vi "Logging Settings Session.vi"(0 "Type":enum16{"Set Settings", "Get Settings"}(ring)=enum."Get Settings", 11 "Error In":errorcluster) -> (6 "Logging Settings":T1={"Logging Interval [s]"=1.0, "Use Lowpass Filter"=TRUE, "Tf [s]"=5.0, "Logging Data to File"=TRUE, "Log Folder"=path "c:/Temp/Data.lvm", "Logging Data to Cloud Service"=FALSE, "Data Cloud Service Url"="http://127.0.0.1:8001/DataWS", "Use Random Data"=TRUE}, 15 "Error Out":errorcluster)   [LabVIEW 2019]
uses:
  Controls/Logging Settings.ctl
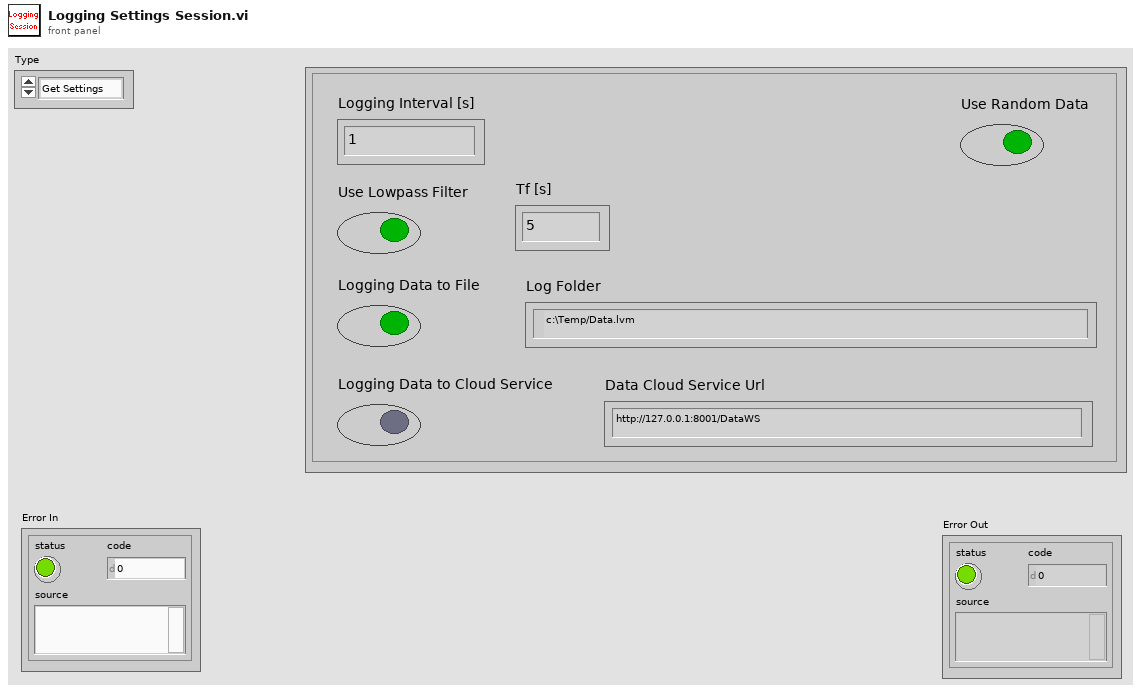
[diagram p1: front panel]
types:
  T1 = typedef "Logging Settings.ctl" = cluster{"Logging Interval [s]":dbl, "Use Lowpass Filter":bool, "Tf [s]":dbl, "Logging Data to File":bool, "Log Folder":path, "Logging Data to Cloud Service":bool, "Data Cloud Service Url":string, "Use Random Data":bool}
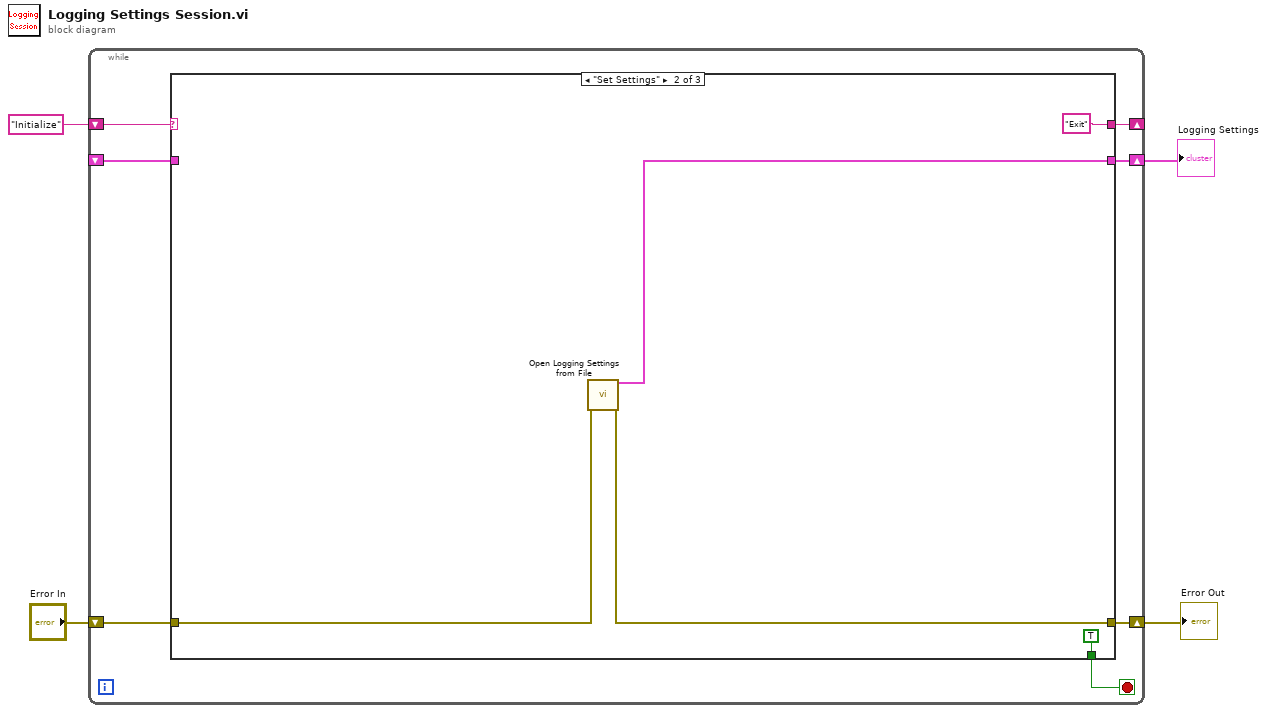
[diagram p0: block diagram]
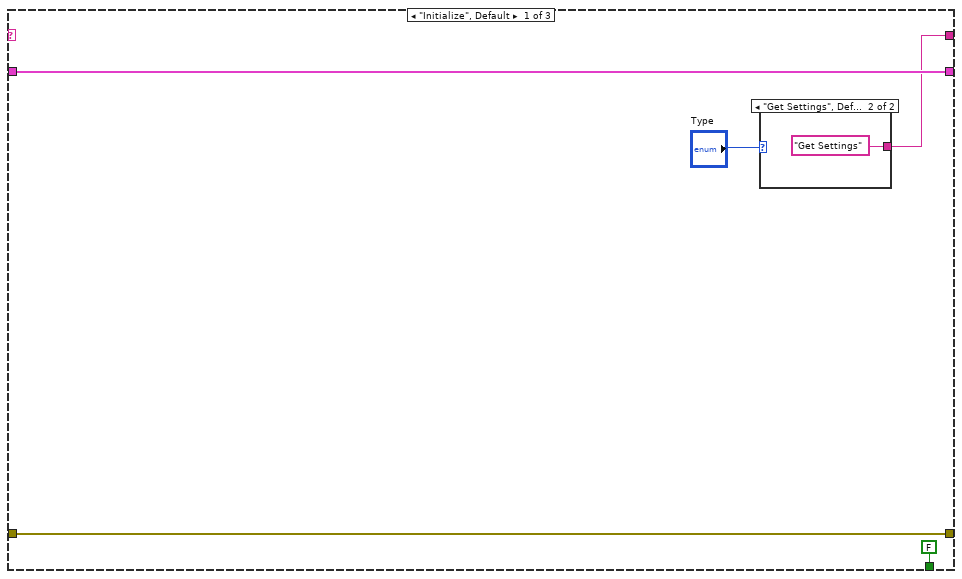
[diagram p2: hidden frame]
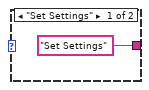
[diagram p3: hidden frame]
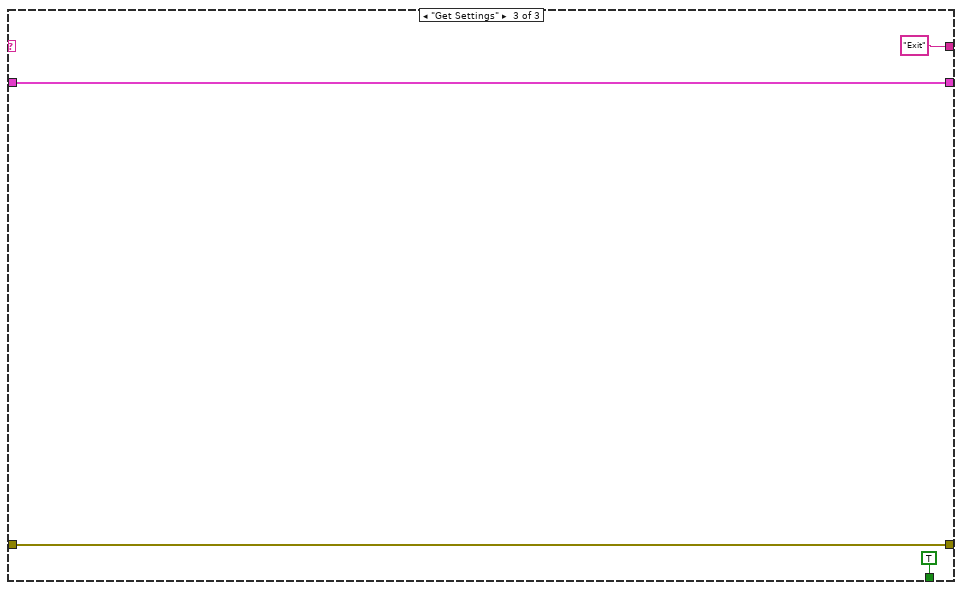
[diagram p4: hidden frame]
diagram:
  n1 = while {
    shift-right: [w6] -> _
    shift-left: "Initialize" ("key") -> [w11]
    shift-right: [w7] -> w1
    shift-left: _ -> [w10]
    shift-right: [w8] -> w2
    shift-left: "Error In" -> [w9]
    stop <- w5 stop-if-true
    n2 = case shown="\"Set Settings\"" w11 {
      tunnel: w10 -> [w14 _ w24]
      tunnel: w9 -> [w15 w20 w25]
      tunnel: [w15 w19 w25] -> w8
      tunnel: [w14 w21 w24] -> w7
      tunnel: [w12 "Exit" ("key") "Exit" ("key")] -> w6
      tunnel: [FALSE TRUE TRUE] -> w5
      frame "Initialize", Default {
        n3 = case shown="\"Get Settings\", Default" "Type" {
          tunnel: ["Set Settings" ("key") "Get Settings" ("key")] -> w12
          frame "Set Settings" {
          }
          frame "Get Settings", Default {
          }
        }
      }
      frame "Set Settings" {
        n4 = call "Open Logging Settings from File.vi"("Error In"=w20) -> ("Logging Settings"=w21:T1, "Error Out"=w19:errorcluster)  [unwired: 13 in]
      }
      frame "Get Settings" {
      }
    }
  }
  "Error Out" <- w2
  "Logging Settings" <- w1
